vi "Untitled 1.vi"() -> ()   [LabVIEW 2017]
panel:
  out "Class Name":string
  in  "Numeric":dbl
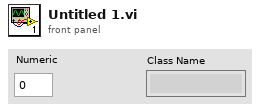
[diagram p1: front panel]
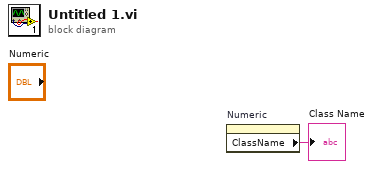
[diagram p0: block diagram]
diagram:
  n1 = property on="Numeric" class="DigNum (strict)"() -> ("ClassName"=→"Class Name":string)  [unwired: 2 in, 2 out]
